vi "Linear Interpolation or Extrapolation.vi"(9 "X":dbl, 10 "Point 2":cluster{"X":dbl, "Y":dbl}, 11 "Point 1":cluster{"X":dbl, "Y":dbl}) -> (3 "Y":dbl)   [LabVIEW 2010]
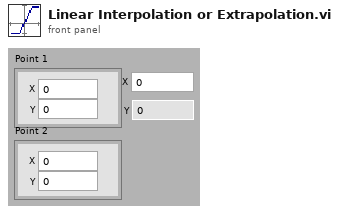
[diagram p1: front panel]
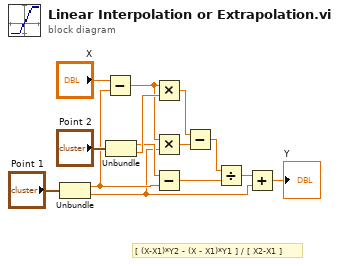
[diagram p0: block diagram]
diagram:
  # "[ (X-X1)*Y2 - (X - X1)*Y1 ] / [ X2-X1 ]"
  n1 = Unbundle("Point 1") -> ("X"=w5:dbl, "Y"=w2:dbl)
  n2 = Subtract(x="X", y=w5) -> (x-y=w10:dbl)
  n3 = Unbundle("Point 2") -> ("X"=w6:dbl, "Y"=w11:dbl)
  n4 = Multiply(x=w10, y=w11) -> (x*y=w9:dbl)
  n5 = Multiply(x=w10, y=w2) -> (x*y=w8:dbl)
  n6 = Subtract(x=w6, y=w5) -> (x-y=w4:dbl)
  n7 = Subtract(x=w9, y=w8) -> (x-y=w7:dbl)
  n8 = Divide(x=w7, y=w4) -> (x/y=w3:dbl)
  n9 = Add(x=w3, y=w2) -> (x+y=→"Y":dbl)
